vi "Evaluate Num Shared Variable.vi"(6 "error in (no error)":errorcluster, 7 "Access":T1=enum."Read", 8 "Read Values":dbl[](array[numeric]), 9 "Num Array Index":i32[](array[numeric]), 10 "Num Array":refnum<k21>[](array[refnum]), 11 "Write Values in":dbl[](array[numeric])) -> (0 "error out":errorcluster, 3 "Write Values out":dbl[](array[numeric]))   [LabVIEW 2015, in "Shared Variable Custom Device.lvlib"]
uses:
  Shared Variable Custom Device.lvlib
  Shared Variable Access.ctl
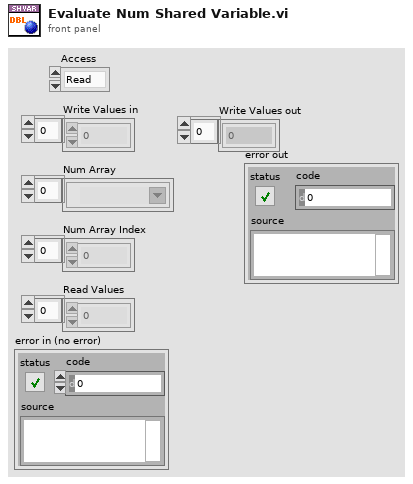
[diagram p1: front panel]
types:
  T1 = typedef "Shared Variable Custom Device.lvlib/Shared Variable Access.ctl" = enum16{"Write", "Read"}
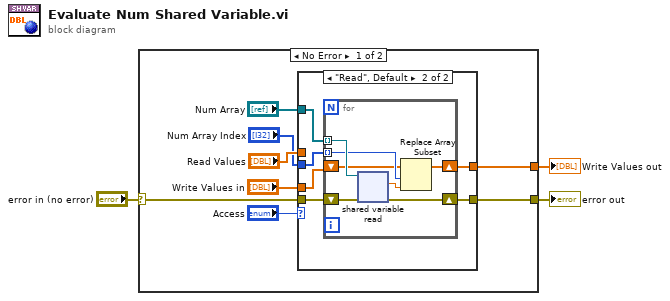
[diagram p0: block diagram]
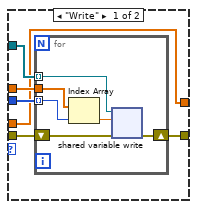
[diagram p2: hidden frame]
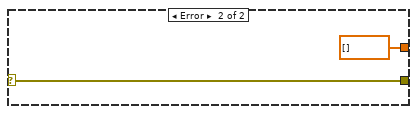
[diagram p3: hidden frame]
diagram:
  n1 = case shown="No Error" "error in (no error)" {
    selector: "error in (no error)" -> [w5 w38]
    tunnel: [w6 w38] -> w3
    tunnel: [w4 dbl[] [] ("Write Values in")] -> w1
    frame No Error {
      n2 = case shown="\"Read\", Default" "Access" {
        tunnel: "Read Values" -> [w17 _]
        tunnel: "Num Array Index" -> [w16 w29]
        tunnel: "Num Array" -> [w15 w28]
        tunnel: "Write Values in" -> [w14 w27]
        tunnel: [w14 w26] -> w4
        tunnel: w5 -> [w13 w25]
        tunnel: [w12 w24] -> w6
        frame "Write" {
          n3 = for {
            tunnel: w15 -> [w23] mode=indexing
            tunnel: w17 -> [w22]
            tunnel: w16 -> [w21] mode=indexing
            shift-right: [w18] -> w12
            shift-left: w13 -> [w19]
            n4 = Index Array(array=w22, index=w21) -> (element=w20:dbl)
            n5 = shared-variable-write(w23, w19, w20) -> (w18:errorcluster)  [unwired: 1 out]
          }
        }
        frame "Read", Default {
          n6 = for {
            tunnel: w28 -> [w36] mode=indexing
            shift-right: [w33] -> w26
            shift-left: w27 -> [w34]
            tunnel: w29 -> [w35] mode=indexing
            shift-right: [w31] -> w24
            shift-left: w25 -> [w30]
            n7 = shared-variable-read(w36, w30) -> (w31:errorcluster, w32:dbl)  [unwired: 2 out]
            n8 = Replace Array Subset(array=w34, new element=w32, index=w35) -> (w33:dbl[])
          }
        }
      }
    }
    frame Error {
    }
  }
  "error out" <- w3
  "Write Values out" <- w1
